vi "AwakeRunnerShock.vi"() -> ()   [LabVIEW 2012]
uses:
  <vilib>/vision/Image Controls.llb/IMAQ Image.ctl
  <vilib>/Instr/_visa.llb/Select Event Type.ctl
  <instrlib>/niHWS/nihws.llb/niHWS Open File Permissions ID.ctl
  <vilib>/DAQmx/write.llb/DAQmx Write (Digital Bool 1Line 1Point).vi
  <vilib>/DAQmx/read.llb/DAQmx Read (Analog Wfm 1Chan NSamp).vi
  <instrlib>/niHWS/nihws.llb/niHWS Write Analog DBL.vi
  <instrlib>/niHWS/nihws.llb/niHWS Write Analog WDT.vi
  <vilib>/DAQmx/miscellaneous.llb/DAQmx Fill In Error Info.vi
  <vilib>/express/express arith-compare/Formula/XNode/ExpressFormulaBlockNode.xnode
  <resource>/objmgr/daqmx.rc
  <vilib>/vision/NI_Vision_Development_Module.lvlib
  <vilib>/ptbypt/NI_PtbyPt.lvlib
panel:
  out "Shock Countdown":dbl
  in  "Random":bool
  in  "shock time (ms)":u32
  in  "Shock Button":bool
  out "Shock":bool
  in  "SyncWrite":bool
  out "Click Value":i8
  out "Image Dst Out":T1
  out "Ephys Rate":dbl=1000.0
  out "Waveform Chart":waveform(dbl)(graph)
  out "Speed History":dbl(graph)
  in  "Magnify":bool
  in  "stop":bool
  out "Camera":T1(plugin-control)
  out "Rec Time":dbl format="%#_3g"
  out "fps":dbl format="%#_2g"
  in  "Rec":bool
  in  "Path":path
  in  "Gain":dbl(slide)=2.6607250597988097 min=1.0 max=3.9810717055349722 scale=0.0..4.0
  in  "Exposure Time":dbl(slide)=16602.0 min=56.0 max=16602.0 scale=0.0..16600.0
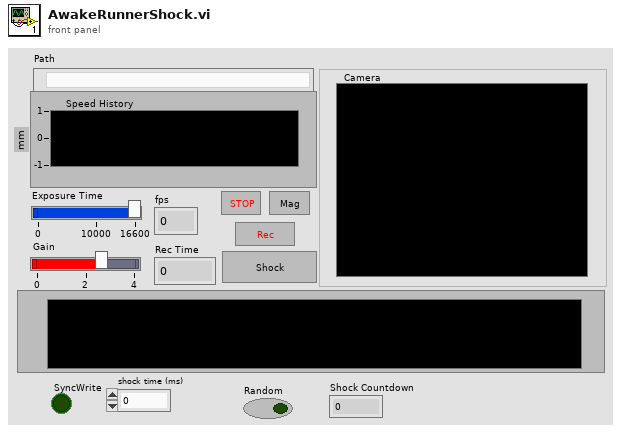
[diagram p1: front panel]
types:
  T1 = typedef "IMAQ Image.ctl" = refnum<image>
  T2 = enum32{"Invalid", "Standard", "Closed", "Hidden", "Minimized", "Maximized"}
  T3 = typedef "niHWS Open File Permissions ID.ctl" = enum32{"Read Only", "Read/Write Existing", "Read/Write/Create New", "Read/Write/Create New Always"}
  T4 = typedef "Select Event Type.ctl" = u32
  T5 = typedef "AviRefnum.ctl" = refnum<k1>
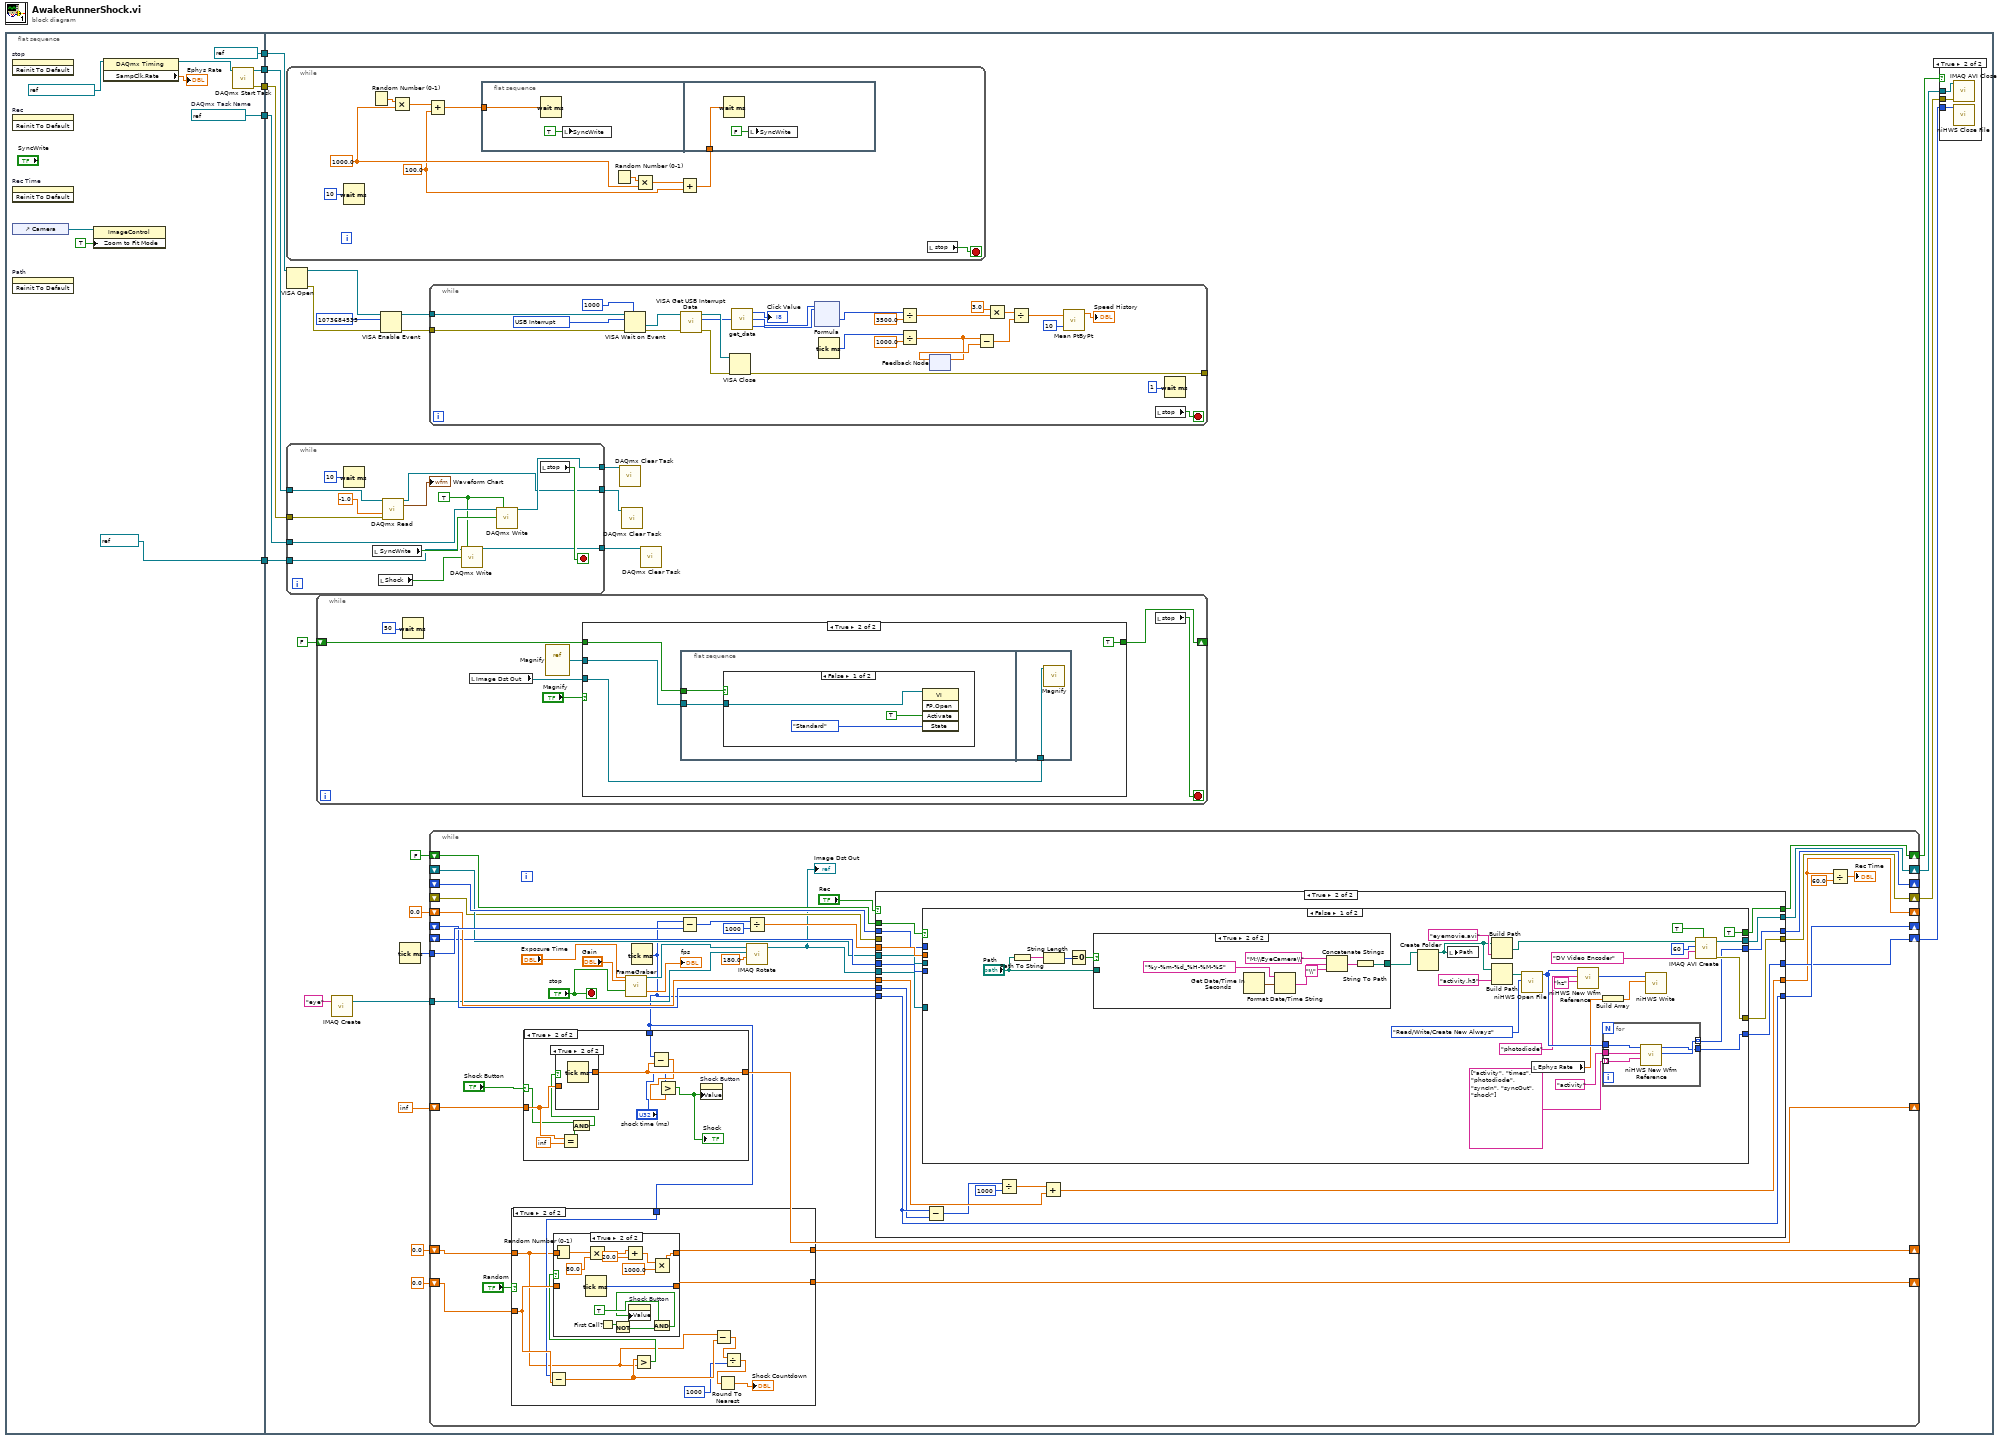
[diagram p0: block diagram]
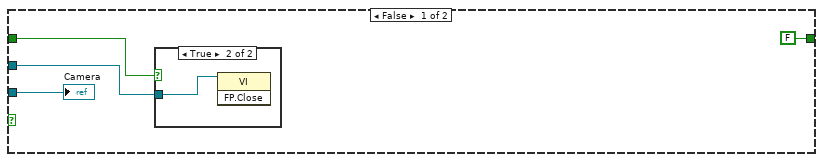
[diagram p2: hidden frame]
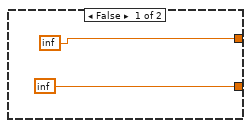
[diagram p6: hidden frame]
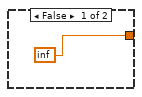
[diagram p8: hidden frame]
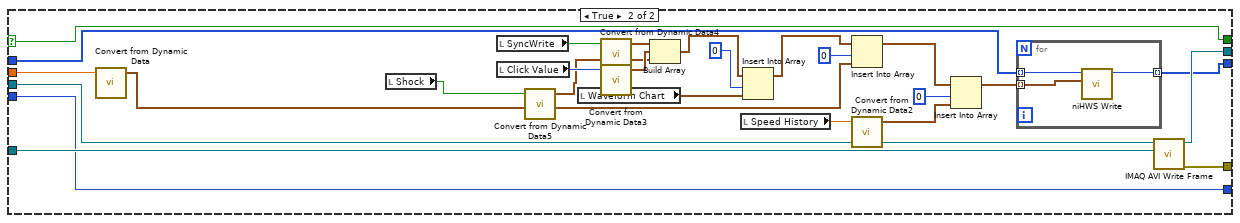
[diagram p12: hidden frame]
diagram:
  n1 = flat-sequence {
    tunnel: [w13] -> w5
    tunnel: [w12] -> w4
    tunnel: [refnum<visa-resource-name> "Mouse2" ("VISA resource name")] -> w3
    tunnel: [w7] -> w2
    tunnel: [refnum<k21> "Shock" ("task/channels in")] -> w1
    tunnel: w5 -> [w33]
    tunnel: w4 -> [w32]
    tunnel: w3 -> [w24]
    tunnel: w2 -> [w23]
    tunnel: w1 -> [w21]
    frame #0 {
      w7 = refnum<k21> "DigitalSync"  # DAQmx Task Name
      n2 = invoke on="stop" class="Bool (strict)" method="Reinit To Default"() -> ()  [unwired: 3 in, 3 out]
      n3 = invoke on="Rec" class="Bool (strict)" method="Reinit To Default"() -> ()  [unwired: 3 in, 3 out]
      n4 = invoke on="Rec Time" class="DigNum (strict)" method="Reinit To Default"() -> ()  [unwired: 3 in, 3 out]
      n5 = control-ref of="Camera"() -> (w15:refnum<vi>)
      n6 = invoke on="Path" class="Path" method="Reinit To Default"() -> ()  [unwired: 3 in, 3 out]
      n7 = property on="Property Node" class="ImageControl"(reference=w15, "Zoom to Fit Mode"=TRUE) -> ()  [unwired: 1 in, 2 out]
      n8 = property class="DAQmx Timing"(reference=refnum<k21> "PhotodiodeBall" ("task/channels in")) -> (reference out=w9:refnum<k21>, "SampClk.Rate"=→"Ephys Rate":dbl)  [unwired: 1 in, 1 out]
      n9 = call <vilib>:"DAQmx Start Task.vi"("task/channels in"=w9) -> ("task out"=w13:refnum<k21>, "error out"=w12:errorcluster)  [unwired: 13 in]
    }
    frame #1 {
      n10 = while {
        stop <- w43 stop-if-true
        w44 = 100.0 ("y")
        w45 = 1000.0 ("y")
        n11 = Wait (ms)(milliseconds to wait=u32 10) -> ()  [unwired: 1 out]
        n12 = Random Number (0-1)() -> (number: 0 to 1=w51:dbl)
        n13 = Multiply(x=w51, y=w45) -> (x*y=w50:dbl)
        n14 = Add(x=w50, y=w44) -> (x+y=w49:dbl)
        n15 = flat-sequence {
          tunnel: w49 -> [w52]
          tunnel: w46 -> [w54]
          frame #0 {
            n16 = Wait (ms)(milliseconds to wait=w52) -> ()  [unwired: 1 out]
            n17 = local write "SyncWrite"(TRUE ("data")) -> ()
          }
          frame #1 {
            n18 = Wait (ms)(milliseconds to wait=w54) -> ()  [unwired: 1 out]
            n19 = local write "SyncWrite"(FALSE ("data")) -> ()
          }
        }
        n20 = Random Number (0-1)() -> (number: 0 to 1=w47:dbl)
        n21 = Multiply(x=w47, y=w45) -> (x*y=w48:dbl)
        n22 = Add(x=w48, y=w44) -> (x+y=w46:dbl)
        n23 = local read "stop"() -> (w43:bool)
      }
      n24 = VISA Open(VISA resource name=w24) -> (VISA resource name=w29:refnum<visa-resource-name>, error out=w28:errorcluster)  [unwired: 1 in, 3 out]
      n25 = while {
        tunnel: w33 -> [w106]
        tunnel: w32 -> [w105]
        tunnel: w23 -> [w101]
        tunnel: [w100] -> w22
        tunnel: w21 -> [w98]
        tunnel: [w97] -> w20
        tunnel: [w96] -> w19
        stop <- w107 stop-if-true
        w95 = TRUE ("auto start")
        n26 = Wait (ms)(milliseconds to wait=u32 10) -> ()  [unwired: 1 out]
        n27 = local read "SyncWrite"() -> (w99:bool)
        n28 = local read "Shock"() -> (w94:bool)
        n29 = call-poly <vilib>:"DAQmx Read.vi"("task/channels in"=w106, "timeout"=-1.0, "error in"=w105) -> ("task out"=w97:refnum<k21>, "data"=→"Waveform Chart":waveform(dbl))  [unwired: 10 in, 1 out]
        n30 = call-poly <vilib>:"DAQmx Write.vi"("task/channels in"=w98, "auto start"=w95, "data"=w94) -> ("task out"=w96:refnum<k21>)  [unwired: 10 in, 2 out]
        n31 = call-poly <vilib>:"DAQmx Write.vi"("task/channels in"=w101, "auto start"=w95, "data"=w99) -> ("task out"=w100:refnum<k21>)  [unwired: 10 in, 2 out]
        n32 = local read "stop"() -> (w107:bool)
      }
      n33 = while {
        shift-right: [w111] -> _
        shift-left: FALSE -> [w110]
        stop <- w112 stop-if-true
        n34 = Wait (ms)(milliseconds to wait=u32 50) -> ()  [unwired: 1 out]
        n35 = local read "Image Dst Out"() -> (w108:T1)
        n36 = vi-ref "Magnify.vi"() -> (w114:refnum<vi>)
        n37 = case shown="True" "Magnify" {
          tunnel: w114 -> [w118 w123]
          tunnel: [FALSE TRUE] -> w111
          tunnel: w110 -> [w117 w121]
          tunnel: w108 -> [w115 w120]
          frame False {
            n38 = case shown="True" w117 {
              tunnel: w118 -> [_ w119]
              frame False {
              }
              frame True {
                n39 = invoke class="VI" method="FP.Close"(reference=w119) -> ()  [unwired: 2 in, 3 out]
              }
            }
            "Camera" <- w115
          }
          frame True {
            n40 = flat-sequence {
              tunnel: w123 -> [w125]
              tunnel: w121 -> [w124]
              tunnel: w120 -> [w129]
              frame #0 {
                n41 = case shown="False" w124 {
                  tunnel: w125 -> [w127 _]
                  frame False {
                    n42 = invoke class="VI" method="FP.Open"(reference=w127, "Activate"=TRUE ("Wait Until Done"), "State"=T2."Standard") -> ()  [unwired: 2 in, 5 out]
                  }
                  frame True {
                  }
                }
              }
              frame #1 {
                n43 = call "Magnify.vi"("Camera 2"=w129) -> ()  [unwired: 11 in]
              }
            }
          }
        }
        n44 = local read "stop"() -> (w112:bool)
      }
      n45 = call "IMAQ Create"("Image Name"="eye") -> ("New Image"=w25:T1)  [unwired: 4 in, 1 out]
      n46 = VISA Enable Event(8:w28, 10:u32 1073684535 ("event type"), 11:w29) -> (0:w31:errorcluster, 3:w30:refnum<visa-resource-name>)  [unwired: 1 out]
      n47 = Tick Count (ms)() -> (millisecond timer value=w38:u32)
      n48 = while {
        tunnel: w30 -> [w83]
        tunnel: [w82] -> _
        tunnel: w31 -> [w75]
        stop <- w76 stop-if-true
        w74 = T4 1073684535 items=["Service Request"=1073684491, "Trigger"=3221168138, "Clear"=1073684493, "VXI Signal"=1073684512, "VXI/VME Interrupt"=3221168161, "VXI/VME Sysfail"=1073684509, "VXI/VME Sysreset"=1073684510, "GPIB CIC"=1073684498, "GPIB Talk"=1073684499, "GPIB Listen"=1073684500, "PXI Interrupt"=1073684514, "Serial Break"=1073684515, "Serial TermChar"=1073684516, "Serial CTS"=1073684521, "Serial DSR"=1073684522, "Serial DCD"=1073684524, "Serial RI"=1073684526, "Serial Character"=1073684533, "USB Interrupt"=1073684535, "All Enabled"=1073709055] ("Event Type")
        n49 = VISA Wait on Event(7:u32 1000 ("timeout (0)"), 8:w75, 10:w74, 11:w83) -> (0:w79:errorcluster, 1:w78:refnum<visa-resource-name>)  [unwired: 3 out]
        n50 = call <vilib>:"VISA Get USB Interrupt Data.vi"("error in (no error)"=w79, "VISA USB Intr Event"=w78) -> ("error out"=w81:errorcluster, "data buffer"=w72:u8[], "VISA USB Intr Event out"=w80:refnum<visa-resource-name>)  [unwired: 7 out]
        n51 = VISA Close(VISA resource name=w80, error in (no error)=w81) -> (error out=w82:errorcluster)
        n52 = call "get_data.vi"("data buffer"=w72) -> ("Click Value"=→"Click Value":i8, "X Value"=w56:i8, "Y Value"=w57:i8)
        n53 = xnode ("Formula")("X1"=w56, "X2"=w57) -> ("Result"=w69:i8)  [unwired: 1 in, 1 out]
        n54 = Tick Count (ms)() -> (millisecond timer value=w67:u32)
        n55 = Divide(x=w69, y=3500.0 ("DPI")) -> (x/y=w64:dbl)
        n56 = Divide(x=w67, y=1000.0) -> (x/y=w65:dbl)
        n57 = feedback #1() -> (w70:dbl)  [unwired: 1 in]
        n58 = feedback-in #1(w65) -> ()
        n59 = Subtract(x=w65, y=w70) -> (x-y=w68:dbl)
        n60 = Multiply(x=3.0, y=w64) -> (x*y=w63:dbl)
        n61 = Divide(x=w63, y=w68) -> (x/y=w60:dbl)
        n62 = call <vilib>:"Mean PtByPt.vi"("x"=w60, "sample length"=10) -> ("mean"=→"Speed History":dbl)  [unwired: 2 in, 1 out]
        n63 = local read "stop"() -> (w76:bool)
        n64 = Wait (ms)(milliseconds to wait=u32 1) -> ()  [unwired: 1 out]
      }
      n65 = while {
        tunnel: w38 -> [w169]
        shift-right: [w168] -> _
        shift-left: _ -> [w167]
        shift-right: [w149] -> _
        shift-left: 0.0 -> [w166]
        shift-right: [w157] -> w36
        shift-left: FALSE -> [w158]
        shift-right: [w154] -> _
        shift-left: _ -> [w153]
        shift-right: [w155] -> w35
        shift-left: _ -> [w152]
        shift-right: [w170] -> w41
        shift-left: _ -> [w151]
        shift-right: [w142] -> w40
        shift-left: _ -> [w150]
        tunnel: w25 -> [w143]
        shift-right: [w140] -> _
        shift-left: inf -> [w139]
        shift-right: [w137] -> _
        shift-left: 0.0 ("millisecond timer value") -> [w135]
        shift-right: [w134] -> _
        shift-left: 0.0 -> [w133]
        stop <- "stop" stop-if-true
        n66 = call "FrameGraber.vi"("Exposure Time"="Exposure Time", "Gain"="Gain", "Stop (F)"="stop") -> ("Image Out"=w146:T1, "Frame Rate"=→"fps":dbl)  [unwired: 20 in, 3 out]
        n67 = Tick Count (ms)() -> (millisecond timer value=w136:u32)
        n68 = case shown="True" "Random" {
          tunnel: [inf w183] -> w137
          tunnel: w136 -> [_ w181]
          tunnel: w135 -> [_ w182]
          tunnel: [inf w179] -> w134
          tunnel: w133 -> [_ w177]
          frame False {
          }
          frame True {
            n69 = Subtract(x=w181, y=w182) -> (x-y=w178:dbl)
            n70 = Greater?(x=w178, y=w177) -> (0:w180:bool)
            n71 = case shown="True" w180 {
              tunnel: [w185 w193] -> w183
              tunnel: [w184 w191] -> w179
              tunnel: w182 -> [w185 _]
              tunnel: w177 -> [w184 _]
              frame False {
              }
              frame True {
                n72 = Random Number (0-1)() -> (number: 0 to 1=w197:dbl)
                n73 = Tick Count (ms)() -> (millisecond timer value=w193:u32)
                n74 = Multiply(x=w197, y=80.0) -> (x*y=w194:dbl)
                n75 = First Call?() -> (First Call?: T/F=w190:bool)
                n76 = Not(x=w190) -> (.not. x?=w188:bool)
                n77 = Add(x=w194, y=20.0) -> (x+y=w192:dbl)
                n78 = Multiply(x=w192, y=1000.0) -> (x*y=w191:dbl)
                n79 = And(x=TRUE ("Shock Button"), y=w188) -> (x .and. y?=w187:bool)
                n80 = property on="Shock Button" class="Bool (strict)"("Value"=w187) -> ()  [unwired: 2 in, 2 out]
              }
            }
            n81 = Subtract(x=w177, y=w178) -> (x-y=w176:dbl)
            n82 = Divide(x=w176, y=1000) -> (x/y=w175:dbl)
            n83 = Round To Nearest(number=w175) -> (nearest integer value=→"Shock Countdown":dbl)
          }
        }
        n84 = case shown="True" "Shock Button" {
          selector: "Shock Button" -> [_ w201]
          tunnel: w136 -> [_ w207]
          tunnel: [inf w208] -> w140
          tunnel: w139 -> [_ w203]
          frame False {
          }
          frame True {
            n85 = Equal?(x=w203, y=inf) -> (x = y?=w202:bool)
            n86 = And(x=w201, y=w202) -> (x .and. y?=w200:bool)
            n87 = case shown="True" w200 {
              tunnel: [w209 w210] -> w208
              tunnel: w203 -> [w209 _]
              frame False {
              }
              frame True {
                n88 = Tick Count (ms)() -> (millisecond timer value=w210:u32)
              }
            }
            n89 = Subtract(x=w207, y=w208) -> (x-y=w206:dbl)
            n90 = Greater?(x="shock time (ms)", y=w206) -> (0:w199:bool)
            "Shock" <- w199
            n91 = property on="Shock Button" class="Bool (strict)"("Value"=w199) -> ()  [unwired: 2 in, 2 out]
          }
        }
        n92 = Subtract(x=w136, y=w169) -> (x-y=w161:u32)
        n93 = Divide(x=w161, y=1000) -> (x/y=w159:dbl)
        n94 = call "IMAQ Rotate"("Angle (degrees)"=sgl 180.0, "Image Dst"=w143, "Image Src"=w146) -> ("Image Dst Out"=w145:T1)  [unwired: 7 in, 1 out]
        "Image Dst Out" <- w145
        n95 = case shown="True" "Rec" {
          tunnel: [w212 w226] -> w170
          tunnel: [w211 w225] -> w142
          tunnel: [w216 w232] -> w149
          tunnel: w159 -> [_ w223]
          tunnel: [w217 w235] -> w168
          tunnel: w136 -> [w217 w235]
          tunnel: w167 -> [_ w234]
          tunnel: w166 -> [w216 w233]
          tunnel: w145 -> [_ w224]
          tunnel: w158 -> [w215 w228]
          tunnel: [w215 w227] -> w157
          tunnel: [w213 w222] -> w155
          tunnel: [w214 w221] -> w154
          tunnel: w153 -> [w214 w220]
          tunnel: w152 -> [w213 w219]
          tunnel: w151 -> [w212 w218]
          tunnel: w150 -> [w211 _]
          frame False {
          }
          frame True {
            n96 = case shown="False" w228 {
              selector: w228 -> [_ w301]
              tunnel: [TRUE w301] -> w227
              tunnel: [w259 w300] -> w226
              tunnel: [w258 w299] -> w225
              tunnel: w224 -> [_ w298]
              tunnel: w223 -> [_ w294]
              tunnel: [w243 w297] -> w222
              tunnel: [w242 w286] -> w221
              tunnel: w220 -> [_ w287]
              tunnel: w219 -> [_ w297]
              tunnel: w218 -> [_ w296]
              frame False {
                n97 = Path To String(path="Path") -> (string=w260:string)
                n98 = String Length(string=w260) -> (length=w261:i32)
                n99 = Equal To 0?(x=w261) -> (x = 0?=w249:bool)
                n100 = case shown="True" w249 {
                  tunnel: [w268 w269] -> w247
                  tunnel: "Path" -> [w268 _]
                  frame False {
                  }
                  frame True {
                    n101 = Get Date/Time In Seconds() -> (seconds since 1Jan1904=w275:timestamp)
                    n102 = Format Date/Time String(time format string (%c)="%y-%m-%d_%H-%M-%S", seconds (now)=w275) -> (date/time string=w272:string)  [unwired: 1 in]
                    n103 = Concatenate Strings("M:\\EyeCamera\\", w272, "\\" ("string")) -> (w270:string)
                    n104 = String To Path(string=w270) -> (path=w269:path)
                  }
                }
                n105 = Create Folder(path (use dialog)=w247) -> (created path=w246:path)  [unwired: 2 in, 2 out]
                n106 = local write "Path"(w246) -> ()
                n107 = Build Path(base path=w246, name or relative path="eyemovie.avi" ("search string")) -> (appended path=w252:path)
                n108 = Build Path(base path=w246, name or relative path="activity.h5" ("search string")) -> (appended path=w250:path)
                n109 = call <instrlib>:"niHWS Open File.vi"("permissions (0:read only)"=niHWS_Open_File_Permissions_ID."Read/Write/Create New Always", "file path"=w250) -> ("file handle"=w241:u32)  [unwired: 8 in, 1 out]
                n110 = local read "Ephys Rate"() -> (w237:dbl)
                n111 = call <instrlib>:"niHWS New Wfm Reference.vi"("waveform name (empty)"="hz", "group name (empty)"="photodiode", "file handle in"=w241) -> ("waveform reference"=w238:u32)  [unwired: 6 in, 2 out]
                n112 = Build Array(w237) -> (w236:dbl[])
                n113 = for {
                  tunnel: w241 -> [w267]
                  tunnel: [w266] -> w242 mode=indexing
                  tunnel: "activity" ("group name (empty)") -> [w265]
                  tunnel: string[] ["activity", "times", "photodiode", "syncIn", "syncOut", "shock"] -> [w264] mode=indexing
                  tunnel: [w263] -> w243
                  n114 = call <instrlib>:"niHWS New Wfm Reference.vi"("waveform name (empty)"=w264, "group name (empty)"=w265, "file handle in"=w267) -> ("waveform reference"=w266:u32, "file handle out"=w263:u32)  [unwired: 6 in, 1 out]
                }
                n115 = call-poly <instrlib>:"niHWS Write.vi"("data"=w236, "waveform reference in"=w238) -> ()  [unwired: 8 in, 2 out]
                n116 = call "IMAQ AVI Create"("Has Data"=TRUE, "Compression Filter"="DV Video Encoder" ("Compressor"), "Frames Per Second"=u32 60, "AVI Path"=w252) -> ("error out"=w258:errorcluster, "Avi Refnum"=w259:T5)  [unwired: 3 in, 3 out]
              }
              frame True {
                n117 = call "Convert from Dynamic Data"("Dynamic Data Type"=w294) -> ("Waveform"=w293:waveform(dbl))  [unwired: 3 in]
                n118 = local read "Shock"() -> (w276:bool)
                n119 = local read "SyncWrite"() -> (w278:bool)
                n120 = local read "Click Value"() -> (w281:i8)
                n121 = call "Convert from Dynamic Data5"("Dynamic Data Type"=w276) -> ("Waveform"=w277:waveform(dbl))  [unwired: 3 in]
                n122 = local read "Waveform Chart"() -> (w283:waveform(dbl))
                n123 = call "Convert from Dynamic Data4"("Dynamic Data Type"=w278) -> ("Waveform"=w279:waveform(dbl))  [unwired: 3 in]
                n124 = call "Convert from Dynamic Data3"("Dynamic Data Type"=w281) -> ("Waveform"=w280:waveform(dbl))  [unwired: 3 in]
                n125 = Build Array(w279, w280, w277) -> (w285:waveform(dbl)[])
                n126 = local read "Speed History"() -> (w290:dbl)
                n127 = Insert Into Array(array=w285, index=0, new element=w283) -> (w282:waveform(dbl)[])
                n128 = Insert Into Array(array=w282, index=0, new element=w293) -> (w291:waveform(dbl)[])
                n129 = call "Convert from Dynamic Data2"("Dynamic Data Type"=w290) -> ("Waveform"=w289:waveform(dbl))  [unwired: 3 in]
                n130 = Insert Into Array(array=w291, index=0, new element=w289) -> (w288:waveform(dbl)[])
                n131 = for {
                  tunnel: w287 -> [w304] mode=indexing
                  tunnel: w288 -> [w303] mode=indexing
                  tunnel: [w302] -> w286 mode=indexing
                  n132 = call-poly <instrlib>:"niHWS Write.vi"("analog waveform"=w303, "waveform reference in"=w304) -> ("waveform reference out"=w302:u32)  [unwired: 8 in, 1 out]
                }
                n133 = call "IMAQ AVI Write Frame"("Image"=w298, "Avi Refnum"=w296) -> ("error out"=w299:errorcluster, "Avi Refnum (duplicate)"=w300:T5)  [unwired: 8 in]
              }
            }
            n134 = Subtract(x=w235, y=w234) -> (x-y=w231:u32)
            n135 = Divide(x=w231, y=1000) -> (x/y=w229:dbl)
            n136 = Add(x=w229, y=w233) -> (x+y=w232:dbl)
          }
        }
        n137 = Divide(x=w149, y=60.0) -> (x/y=→"Rec Time":dbl)
      }
      n138 = call <vilib>:"DAQmx Clear Task.vi"("task in"=w22) -> ()  [unwired: 14 in, 1 out]
      n139 = call <vilib>:"DAQmx Clear Task.vi"("task in"=w20) -> ()  [unwired: 14 in, 1 out]
      n140 = call <vilib>:"DAQmx Clear Task.vi"("task in"=w19) -> ()  [unwired: 14 in, 1 out]
      n141 = case shown="True" w36 {
        tunnel: w41 -> [_ w132]
        tunnel: w40 -> [_ w131]
        tunnel: w35 -> [_ w130]
        frame False {
        }
        frame True {
          n142 = call "IMAQ AVI Close"("error in (no error)"=w131, "Avi Refnum"=w132) -> ()  [unwired: 9 in, 1 out]
          n143 = call <instrlib>:"niHWS Close File.vi"("file handle"=w130) -> ()  [unwired: 10 in, 1 out]
        }
      }
    }
  }
